vi "АЛУ.vi"(3 "Func":T2, 4 "B":T3, 5 "A":T4) -> (0 "Type":bool, 1 "C":bool, 2 "Result":T1)   [LabVIEW 2017]
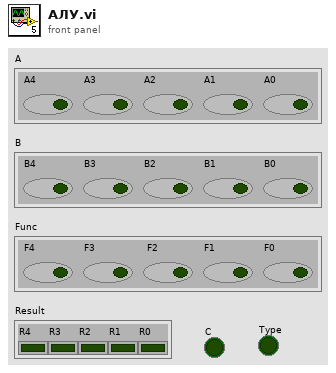
[diagram p1: front panel]
types:
  T1 = cluster{"R4":bool, "R3":bool, "R2":bool, "R1":bool, "R0":bool}
  T2 = cluster{"F4":bool, "F3":bool, "F2":bool, "F1":bool, "F0":bool}
  T3 = cluster{"B4":bool, "B3":bool, "B2":bool, "B1":bool, "B0":bool}
  T4 = cluster{"A4":bool, "A3":bool, "A2":bool, "A1":bool, "A0":bool}
  T5 = cluster{"R4":bool, " R3":bool, " R2":bool, " R1":bool, " R0":bool}
  T6 = cluster{"Y4":bool, "Y3":bool, "Y2":bool, "Y1":bool, "Y0":bool}
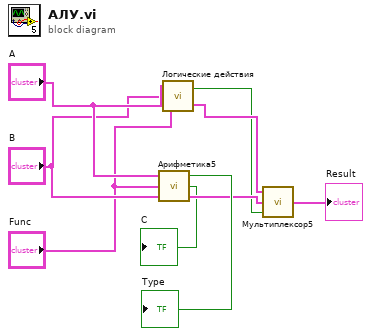
[diagram p0: block diagram]
diagram:
  n1 = call "Арифметика5.vi"("B"="B", "Func"="Func", "A"="A") -> ("Result"=w7:T1, "C"=→"C":bool, "Type"=→"Type":bool)
  n2 = call "Логические действия.vi"("Fun"="Func", "B"="B", "A"="A") -> ("Cluster"=w2:T5, "Plus/min"=w1:bool)
  n3 = call "Мультиплексор5.vi"("C"=w1, "X1"=w7, "X0"=w2) -> ("Y"=→"Result":T6)
